vi "Actor Core.vi"(8 "error in":errorcluster, 11 "Main Window in":refnum<class "Main Window.lvclass">) -> (0 "error out":errorcluster, 3 "Actor out":refnum<class "Actor.lvclass">)   [LabVIEW 2023, in "Main Window.lvlib" / "Main Window.lvclass"]
doc: "(<B>Filename</B>: Actor Framework.lvlib:Actor.lvclass:Actor Core.vi)\n\nReceives messages to the actor, reacts to them, and initiates any error handling that may shut the actor down.\n\nDescendant classes may override this VI to append parallel tasks for the actor to complete while it handles messages. Overrides use the Call Parent Method node."
uses:
  Main Window.lvclass
  C:/Program Files/National Instruments/LabVIEW 2023/vi.lib/ActorFramework/Actor/Actor.lvclass
  <vilib>/ActorFramework/Actor/Actor.lvclass
  Resources/Type Defs/Camera Settings.ctl
  Application/Mode.ctl
  Resources/Type Defs/Movie auto-numbering.ctl
  Main Window.lvclass/Main Window.ctl
  <vilib>/ActorFramework/Actor/Actor.lvclass/Actor.ctl
  <vilib>/ActorFramework/Message Enqueuer/Message Enqueuer.lvclass/Message Enqueuer.ctl
  Application Messages/Stop Live Mode Msg/Stop Live Mode Msg.lvclass/Stop Live Mode Msg.ctl
  Application Messages/Set Enabled Cameras Msg/Set Enabled Cameras Msg.lvclass/Set Enabled Cameras Msg.ctl
  Application Messages/Start Live Mode Msg/Start Live Mode Msg.lvclass/Start Live Mode Msg.ctl
  Application Messages/Open Shutter Msg/Open Shutter Msg.lvclass/Open Shutter Msg.ctl
  Hardware/Microscope/ti2lv/ti2_lightPath.ctl
  Application Messages/Set Detection Msg/Set Detection Msg.lvclass/Set Detection Msg.ctl
  Application Messages/Stage Forward Msg/Stage Forward Msg.lvclass/Stage Forward Msg.ctl
  Application Messages/Photobleach Custom Msg/Photobleach Custom Msg.lvclass/Photobleach Custom Msg.ctl
  Application Messages/Set Laser Power Msg/Set Laser Power Msg.lvclass/Set Laser Power Msg.ctl
  Resources/Type Defs/Movie Series.ctl
  Application Messages/Start Recording Msg/Start Recording Msg.lvclass/Start Recording Msg.ctl
  Application Messages/Start Autofocus Msg/Start Autofocus Msg.lvclass/Start Autofocus Msg.ctl
  Application Messages/Stage Enforce Limits Msg/Stage Enforce Limits Msg.lvclass/Stage Enforce Limits Msg.ctl
  <vilib>/ActorFramework/Message Enqueuer/Enqueue.vi
  Application Messages/Shut Down Msg/Shut Down Msg.lvclass
  C:/Program Files/National Instruments/LabVIEW 2023/vi.lib/ActorFramework/Message/Message.lvclass
  Application Messages/Stop Live Mode Msg/Stop Live Mode Msg.lvclass
  Application Messages/Set Enabled Cameras Msg/Set Enabled Cameras Msg.lvclass
  Application Messages/Start Live Mode Msg/Start Live Mode Msg.lvclass
  Application Messages/Close Shutter Msg/Close Shutter Msg.lvclass
  Application Messages/Open Shutter Msg/Open Shutter Msg.lvclass
  Application Messages/Set Detection Msg/Set Detection Msg.lvclass
  Application Messages/Stage Forward Msg/Stage Forward Msg.lvclass
  Application Messages/Stage Back Msg/Stage Back Msg.lvclass
  Application Messages/Stage Next Lane Msg/Stage Next Lane Msg.lvclass
  Application Messages/Stage Previous Lane Msg/Stage Previous Lane Msg.lvclass
  Application Messages/Photobleach Custom Msg/Photobleach Custom Msg.lvclass
  Application Messages/Stage Move Home Msg/Stage Move Home Msg.lvclass
  Application Messages/Stage Set Home Msg/Stage Set Home Msg.lvclass
  Application Messages/Stage Abort Motion Msg/Stage Abort Motion Msg.lvclass
  Application Messages/Set Laser Power Msg/Set Laser Power Msg.lvclass
  Application Messages/Start Recording Msg/Start Recording Msg.lvclass
  Application Messages/Record Button Off Msg/Cancel Operation Msg.lvclass
  Application Messages/Start Autofocus Msg/Start Autofocus Msg.lvclass
  Application Messages/Stage Enforce Limits Msg/Stage Enforce Limits Msg.lvclass
  Application Messages/Calibrate Polarizer Msg/Calibrate Polarizer Msg.lvclass
  Resources/GLOBAL/GLOBAL Time-critical.vi
  <vilib>/ActorFramework/Message Priority Queue/Priority Enqueue.vi
  Resources/GLOBAL/GLOBAL Debug.vi
  <vilib>/Platform/browser.llb/Open URL in Default Browser (string).vi
  UI Window/UI Window.lvclass
  Hardware/Microscope/ti2lv/ti2lv.lvlib
  C:/FlashGordon/Development/User Interface/UI Window/UI Window.lvclass
  C:/FlashGordon/Development/User Interface/Main Window/Main Window.lvclass
  Application/Application.lvlib
panel:
  in  "Auto-Advance":bool
  out "LaserEnabled":bool[](array[boolean])
  out "current settings":T1={"Exposure Time (ms)"=100.0, "Binning"=enum."2x2", "Scan Mode"=-1, "Frames to Acquire"=1000.0, "Pixel Correction"=FALSE, "Frames to Skip"=1, "File Path"=path "", "Duty cycle"=1.0, "ALEX"=FALSE, "Shutter Enable"=[FALSE, TRUE, FALSE, FALSE], "fluidics trigger frame"=0, "Bit Depth"=15, "Image Width (px)"=0, "Image Height (px)"=0, "Horizontal Offset (px)"=0, "Vertical Offset (px)"=0} {"fluidics trigger frame" max=60000 step=1; "Exposure Time (ms)" min=1.0 max=10000.0 step=1.0}
  out "Saving movie":u8(slide) scale=0.0..100.0
  in  "Stop Button":bool
  in  "Tab Control":enum32{"Imaging", "Advanced"}(tab)
  in  "Stage Position":enum32{"Page 1"}(tab)
  out "Stage Map":picture
  in  "Stop Stage":bool
  in  "Set Home":bool
  in  "Go Home":bool
  in  "Move Forward Button":bool
  in  "Move Back Button":bool
  in  "Next Lane Button":bool
  in  "Previous Lane Button":bool
  in  "Photobleach Button":bool
  in  "Camera Settings":enum32{"Page 1"}(tab)
  in  "frame interval unit":u32(ring)=1 items=["ms"=1, "s"=1000, "min"=60000]
  in  "Use Live Exposure":bool
  in  "Live Exposure Time":dbl=200.0 min=1.0 max=1000.0 step=1.0
  in  "Acquisition Period":dbl=10.0 min=0.1 max=10000.0
  in  "Exposure (ms)":dbl=10.0 min=0.1 max=1000.0 step=1.0
  in  "Illumination:":T2(ring)
  in  "Stream Acquisition":enum32{"Page 1"}(tab)
  in  "Lanes:":i32=1 min=1 max=100 step=1
  in  "Fields:":i32=1 min=1 max=100 step=1
  in  "Frames:":dbl=1000.0 min=10.0
  in  "File Path:":path=path "E:/"
  in  "File Name:":string="Stack"
  in  "Acquisition type":T3=enum."Movie series"
  in  "Injection Countdown":bool
  in  "Auto-Focus":bool
  in  "Microscope Settings":enum32{"Page 1"}(tab)
  out "Measured Power:":string
  in  "Detection":u16(ring)=1 items=["Disabled"]
  in  "Active Shutter Button":bool
  in  "Excitation":T4(array[cluster])=[{"Enable"=FALSE, "Name"="Cy2 (473 nm)", "Power"=0.0}, {"Enable"=TRUE, "Name"="Cy3 (532 nm)", "Power"=0.0}, {"Enable"=FALSE, "Name"="Cy5 (640 nm)", "Power"=0.0}, {"Enable"=FALSE, "Name"="Cy7 (721 nm)", "Power"=0.0}]
  in  "Live Viewer Start":bool
  in  "Cancel Movie Button":bool
  in  "Record Movie Button":bool
  in  "Fluidics Settings":enum32{"Page 1"}(tab)
  in  "Trigger on frame number\n(set to zero to disable)":u16
  in  "Advanced Stage Settings":enum32{"Page 1"}(tab)
  in  "Lane separation (mm)":dbl min=0.0 step=0.001
  in  "Forward step (mm)":dbl min=0.0 step=0.001
  in  "Auto-focus":bool
  in  "Enforce software stage limits":bool=TRUE
  in  "Advanced Illumination Settings":enum32{"Page 2"}(tab)
  out "Duty Cycle:":dbl=0.5 min=0.0 max=1.0 step=0.01 format="%#.3g"
  in  "Calibrate Polarizer":bool
  out "Max shutter rate (Hz)":dbl
  in  "Advanced Camera Settings":enum32{"Page 1"}(tab) caption="Tab Control 2"
  in  "Readout Mode":i32(ring)=-1 items=["Auto"=-1]
  in  "Binning":enum16{"1x1", "2x2", "4x4"}(ring)=enum."2x2"
  in  "Discard First Frames":u32=1
  in  "Pixel Correction":enum16{"Live Only", "On", "Off"}(ring)
  in  "Active Cameras":cluster{"Enable":bool, "Name":string}[](array[cluster])
  out "Current Application Mode":T5
  # "Power (mW)"
  # "(Default = 1)"
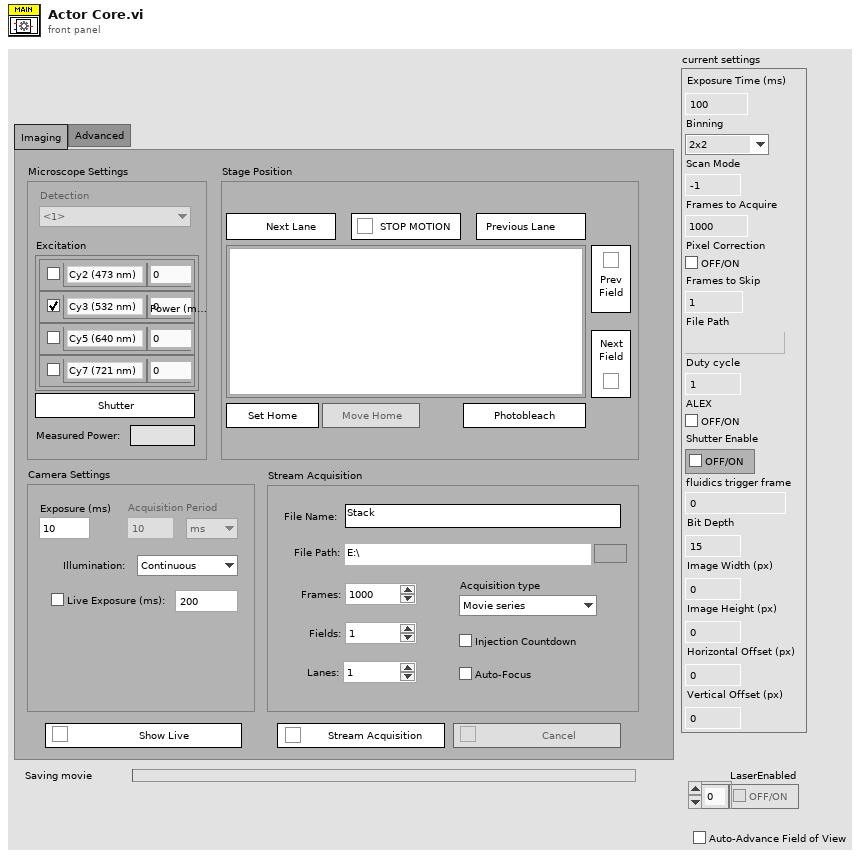
[diagram p1: front panel]
types:
  T1 = typedef "Camera Settings.ctl" = cluster{"Exposure Time (ms)":dbl, "Binning":enum16{"1x1", "2x2", "4x4"}, "Scan Mode":i32, "Frames to Acquire":dbl, "Pixel Correction":bool, "Frames to Skip":u32, "File Path":path, "Duty cycle":dbl, "ALEX":bool, "Shutter Enable":bool[], "fluidics trigger frame":u16, "Bit Depth":u16, "Image Width (px)":u16, "Image Height (px)":u16, "Horizontal Offset (px)":u16, "Vertical Offset (px)":u16}
  T2 = enum16{"Continuous", "Stroboscopic", "Alternating"}
  T3 = typedef "Movie auto-numbering.ctl" = enum16{"Single movie", "Movie series", "Multi-lane series"}
  T4 = cluster{"Enable":bool, "Name":string, "Power":dbl}[]
  T5 = typedef "Application.lvlib/Mode.ctl" = enum16{"Idle", "Cancel", "Live", "Stream", "Autofocus", "Z-Stack"}
  T6 = enum8{"Enabled", "Disabled", "Disabled and Grayed Out"}
  T7 = enum16{"Disable", "Laser Quantum", "Coherent OBIS", "PRM1-Z8", "Coherent HOPS"}
  T8 = typedef "Sync Device Type.ctl" = enum16{"Disabled", "NI DAQ", "Arduino DAQ"}
  T9 = typedef "Physical Camera Assignment.ctl" = cluster{"Channel Name":string, "Serial Number":string, "Flip Vertically":bool, "Flip Horizontally":bool, "wavelength":i16, "photonsPerCount":dbl[]}
  T10 = typedef "Shutter Configuration.ctl" = cluster{"IO Line":tag, "Name":string, "Wavelength":u16, "Max rate (Hz)":dbl}
  T11 = cluster{"Name":string, "Filter Position":u16, "Optical Path":u16}[]
  T12 = typedef "Microscope Type.ctl" = enum16{"Disable", "TE2000", "Eclipse Ti", "Ti2"}
  T13 = enum16{"Disabled", "ESP301", "Ti2", "Ludl", "ASI"}
  T14 = typedef "Laser Configuration.ctl" = cluster{"Serial Port":refnum<visa-resource-name>, "Laser Type":enum16{"Disable", "Laser Quantum", "Coherent OBIS", "PRM1-Z8", "Coherent HOPS", "Cobolt"}, "Polarizer Amplitude":dbl, "Polarizer Theta Zero":dbl, "Wavelength":u16}
  T15 = enum16{"Disable", "Laser Quantum", "Coherent OBIS", "PRM1-Z8", "Coherent HOPS", "Cobolt"}
  T16 = cluster{"Enable":bool, "Name":string, "Power":dbl}
  T17 = typedef "Movie Series.ctl" = cluster{"Camera Settings":T1, "Auto-Advance":bool, "Auto Focus":bool, "Injection Countdown":bool, "Fields":i32, "Lanes":i32, "Acquisition type":T3}
  T18 = typedef "ti2lv.lvlib/ti2_lightPath.ctl" = i32
  T19 = cluster{"Name":string, "Filter Position":u16, "Optical Path":u16}
  T20 = enum16{"Left Button", "Center Button", "Right Button", "Window Close"}
  T21 = cluster{"Enable":bool, "Name":bool, "Power":bool}[]
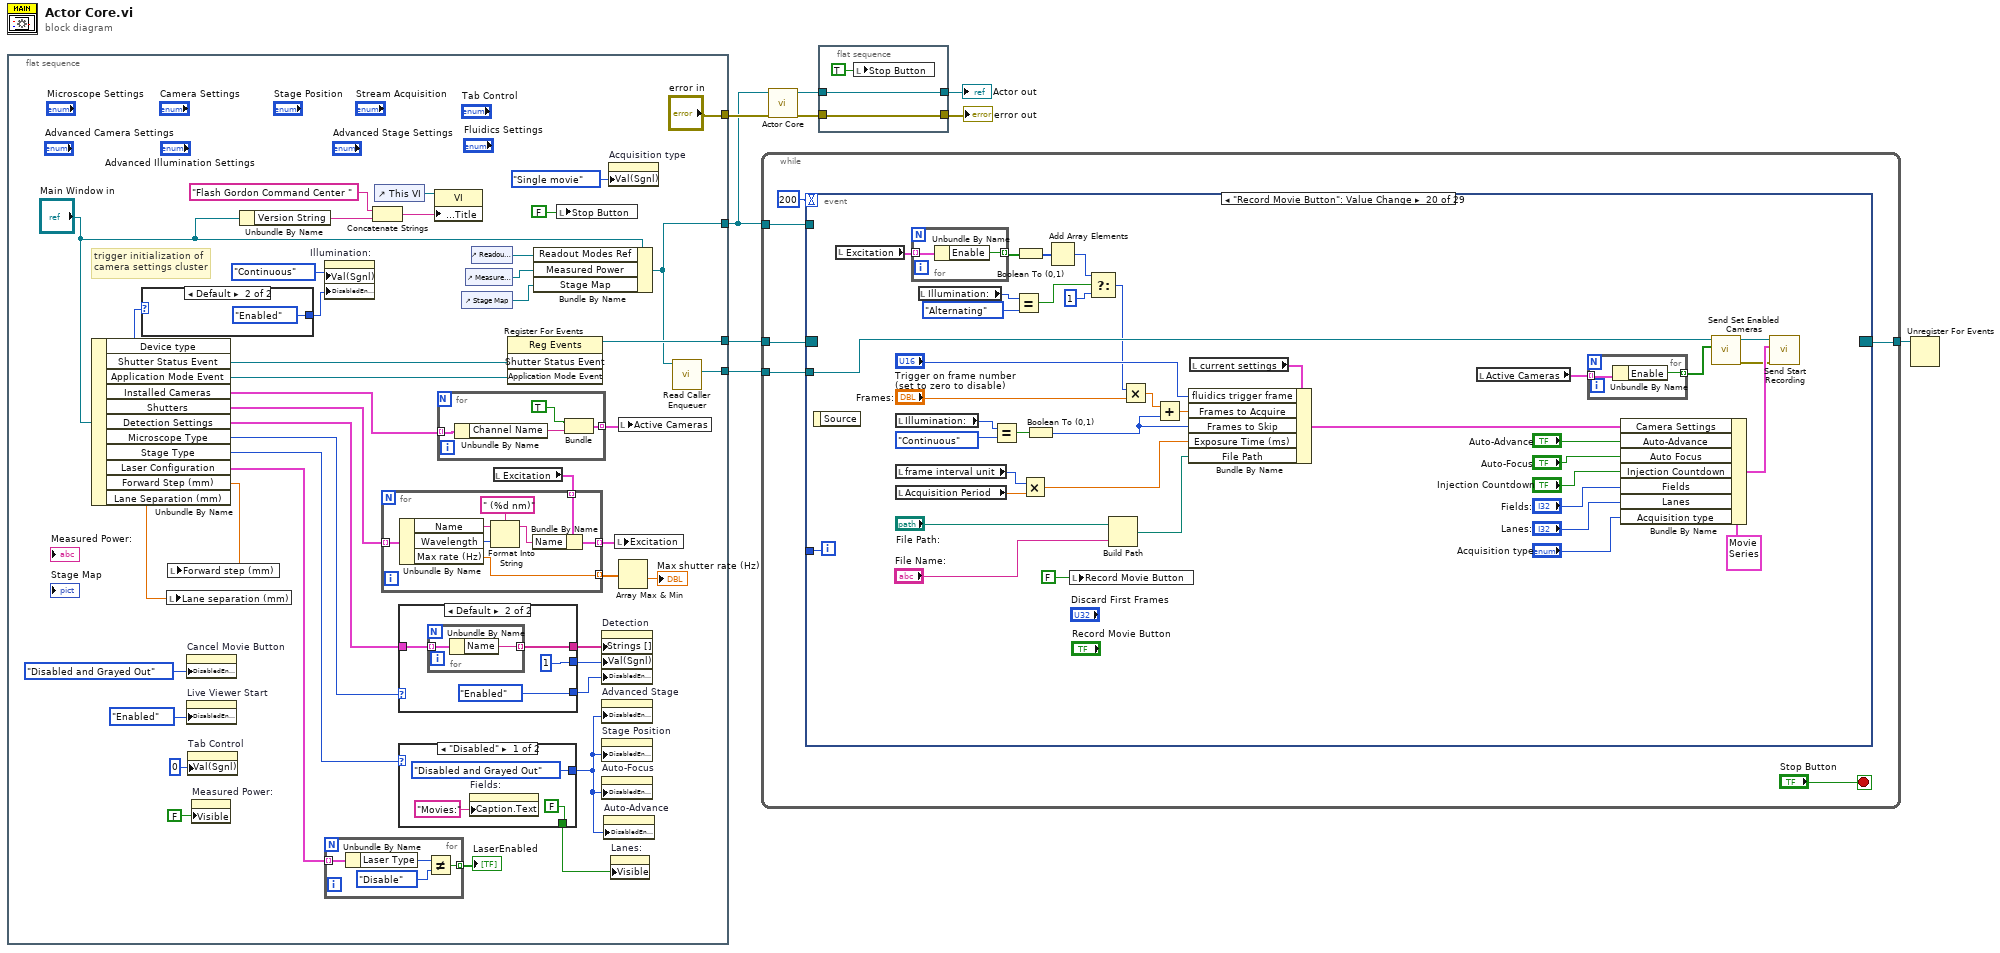
[diagram p0: block diagram]
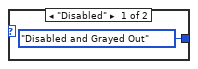
[diagram p2: hidden frame]
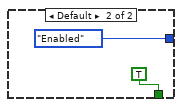
[diagram p3: hidden frame]
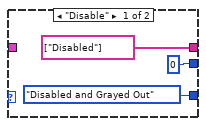
[diagram p4: hidden frame]
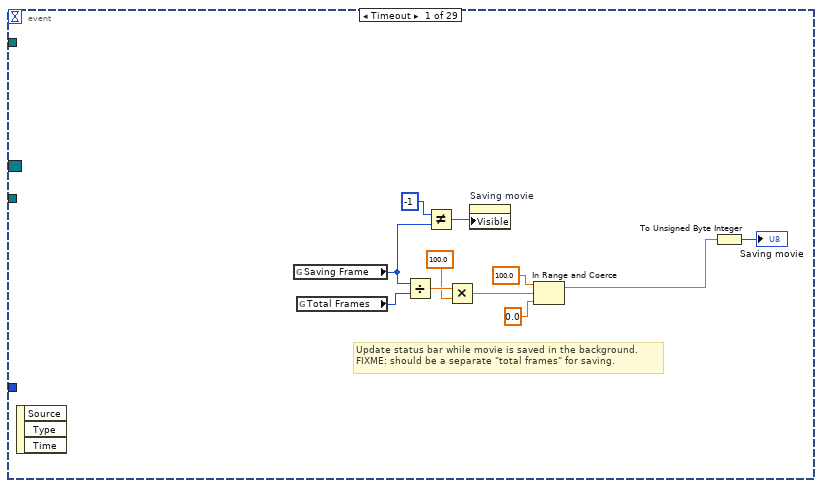
[diagram p5: hidden frame]
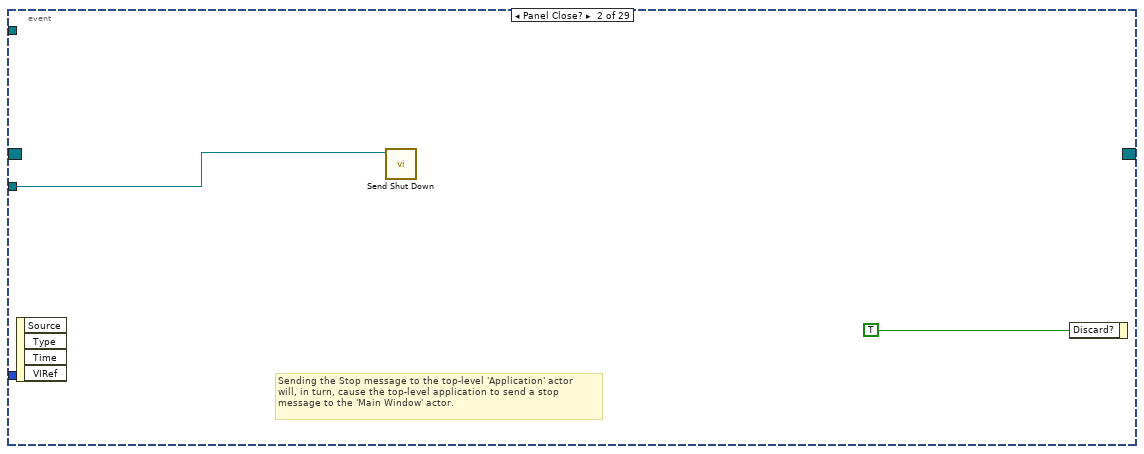
[diagram p6: hidden frame]
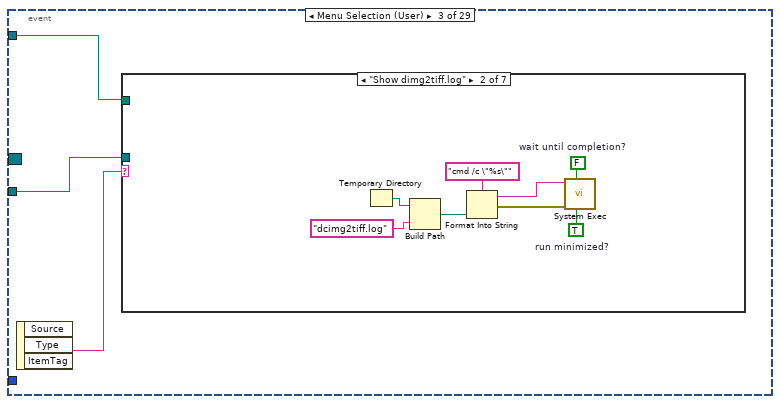
[diagram p7: hidden frame]
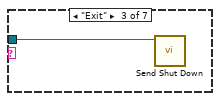
[diagram p9: hidden frame]
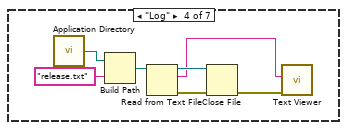
[diagram p10: hidden frame]
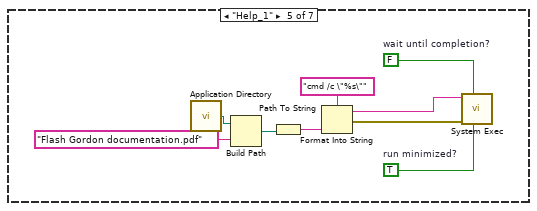
[diagram p11: hidden frame]
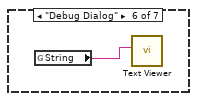
[diagram p12: hidden frame]
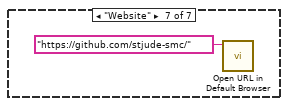
[diagram p13: hidden frame]
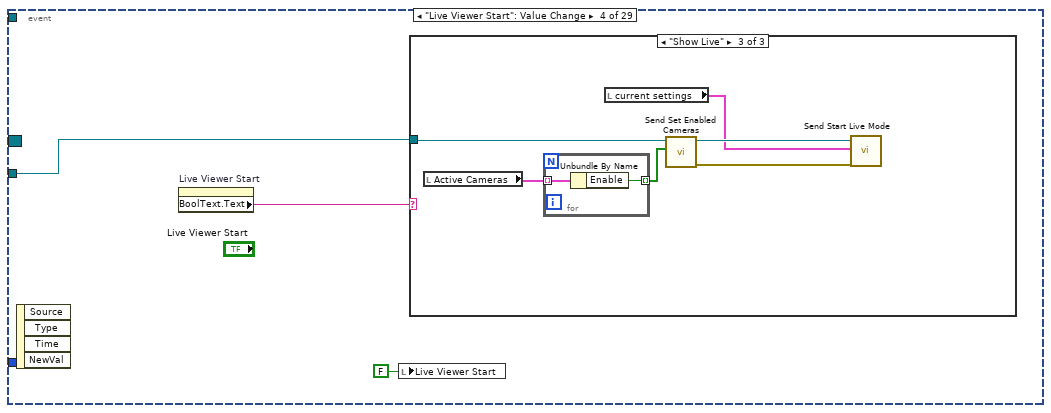
[diagram p14: hidden frame]
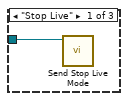
[diagram p15: hidden frame]
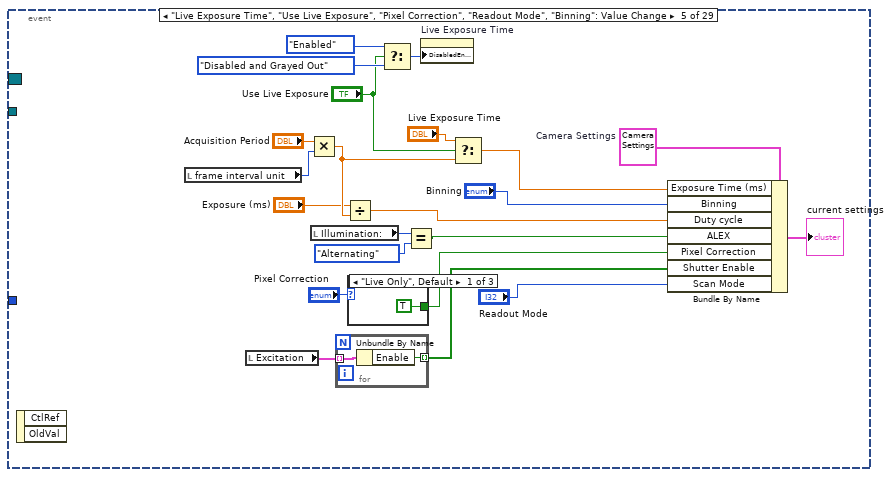
[diagram p17: hidden frame]
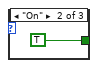
[diagram p18: hidden frame]
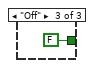
[diagram p19: hidden frame]
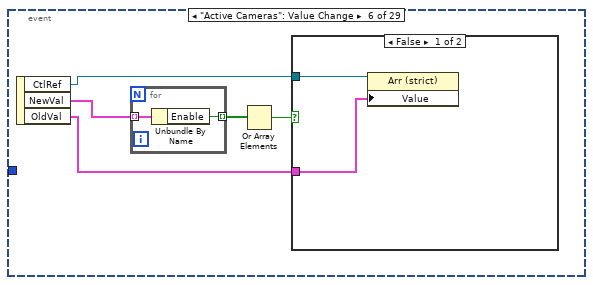
[diagram p20: hidden frame]
diagram:
  n1 = flat-sequence {
    tunnel: [w28] -> w7
    tunnel: ["error in"] -> w8
    tunnel: [w42] -> w6
    tunnel: [w41] -> w5
    frame #0 {
      # "trigger initialization of\ncamera settings cluster"
      n2 = Unbundle By Name("Main Window in") -> ("Device type"=w16:T8, "Shutter Status Event"=w32:refnum<user-event>, "Application Mode Event"=w35:refnum<user-event>, "Installed Cameras"=w23:T9[], "Shutters"=w24:T10[], "Detection Settings"=w37:T11, "Microscope Type"=w40:T12, "Stage Type"=w25:T13, "Laser Configuration"=w20:T14[], "Forward Step (mm)"=w14:dbl, "Lane Separation (mm)"=w13:dbl)
      n3 = case shown="Default" w16 {
        tunnel: [T6."Disabled and Grayed Out" ("Disabled") T6."Enabled" ("Disabled")] -> w15
        frame "Disabled" {
        }
        frame Default {
        }
      }
      n4 = local write "Lane separation (mm)"(w13) -> ()
      n5 = local write "Forward step (mm)"(w14) -> ()
      n6 = property on="Cancel Movie Button" class="Bool (strict)"("DisabledEnum"=T6."Disabled and Grayed Out" ("Disabled")) -> ()  [unwired: 2 in, 2 out]
      n7 = property on="Live Viewer Start" class="Bool (strict)"("DisabledEnum"=T6."Enabled" ("Disabled")) -> ()  [unwired: 2 in, 2 out]
      n8 = property on="Tab Control" class="TabCtl (strict)"("Val(Sgnl)"=0) -> ()  [unwired: 2 in, 2 out]
      n9 = property on="Measured Power:" class="Str"("Visible"=FALSE) -> ()  [unwired: 2 in, 2 out]
      n10 = Unbundle By Name("Main Window in") -> ("Version String"=w47:string)
      n11 = property on="Illumination:" class="Enum (strict)"("Val(Sgnl)"=T2."Continuous" ("Value (Signaling)"), "DisabledEnum"=w15) -> ()  [unwired: 2 in, 2 out]
      n12 = for {
        tunnel: w20 -> [w57] mode=indexing
        tunnel: [w55] -> w19 mode=indexing
        n13 = Unbundle By Name(w57) -> ("Laser Type"=w56:T15)
        n14 = Not Equal?(x=w56, y=T7."Disable") -> (x != y?=w55:bool)
      }
      "LaserEnabled" <- w19
      n15 = Concatenate Strings("Flash Gordon Command Center " ("Front Panel Window:Title"), w47) -> (w48:string)
      n16 = control-ref of="This VI"() -> (w49:refnum<vi>)
      n17 = case shown="Default" w40 {
        tunnel: [T6."Disabled and Grayed Out" ("Disabled") T6."Enabled" ("Disabled")] -> w39
        tunnel: [string[] ["Disabled"] w68] -> w38
        tunnel: w37 -> [_ w67]
        tunnel: [u16 0 u16 1] -> w36
        frame "Disable" {
        }
        frame Default {
          n18 = for {
            tunnel: w67 -> [w71] mode=indexing
            tunnel: [w70] -> w68 mode=indexing
            n19 = Unbundle By Name(w71) -> ("Name"=w70:string)
          }
        }
      }
      n20 = case shown="\"Disabled\"" w25 {
        tunnel: [T6."Disabled and Grayed Out" ("Disabled") T6."Enabled" ("Disabled")] -> w12
        tunnel: [FALSE TRUE] -> w11
        frame "Disabled" {
          n21 = property on="Fields:" class="DigNum (strict)"("Caption.Text"="Movies:") -> ()  [unwired: 2 in, 2 out]
        }
        frame Default {
        }
      }
      n22 = property class="VI"(reference=w49, "Front Panel.Title"=w48) -> ()  [unwired: 1 in, 2 out]
      n23 = for {
        tunnel: w23 -> [w83] mode=indexing
        tunnel: [w81] -> w30 mode=indexing
        n24 = Unbundle By Name(w83) -> ("Channel Name"=w82:string)
        n25 = Bundle(TRUE, "Channel Name"=w82) -> (w81:cluster{bool, "Channel Name":string})  [unwired: 1 in]
      }
      n26 = control-ref of="Stage Map"() -> (w17:refnum<vi>)
      n27 = control-ref of="Measured Power:"() -> (w18:refnum<vi>)
      n28 = control-ref of="Readout Mode"() -> (w26:refnum<vi>)
      n29 = local read "Excitation"() -> (w33:T4)
      n30 = for {
        tunnel: w24 -> [w79] mode=indexing
        tunnel: w33 -> [w75] mode=indexing
        tunnel: [w73] -> w43 mode=indexing
        tunnel: [w72] -> w22 mode=indexing
        n31 = Unbundle By Name(w79) -> ("Name"=w78:string, "Wavelength"=w77:u16, "Max rate (Hz)"=w72:dbl)
        n32 = Format Into String(format string=" (%d nm)", initial string=w78, w77) -> (resulting string=w74:string)  [unwired: 1 in, 1 out]
        n33 = Bundle By Name(cluster=w75, "Name"=w74) -> (w73:T16)
      }
      n34 = register-events(w32, w35) -> (reference out=w42:refnum<event-registration>)  [unwired: 2 in, 1 out]
      n35 = Bundle By Name(cluster="Main Window in", "Readout Modes Ref"=w26, "Measured Power"=w18, "Stage Map"=w17) -> (w28:refnum<class "Main Window.lvclass">)
      n36 = local write "Stop Button"(FALSE ("Stop Button")) -> ()
      n37 = property on="Detection" class="Ring (strict)"("Strings []"=w38, "Val(Sgnl)"=w36, "DisabledEnum"=w39) -> ()  [unwired: 2 in, 2 out]
      n38 = property on="Advanced Stage" class="TabCtl (strict)"("DisabledEnum"=w12) -> ()  [unwired: 2 in, 2 out]
      n39 = property on="Stage Position" class="TabCtl (strict)"("DisabledEnum"=w12) -> ()  [unwired: 2 in, 2 out]
      n40 = property on="Auto-Focus" class="Bool (strict)"("DisabledEnum"=w12) -> ()  [unwired: 2 in, 2 out]
      n41 = property on="Auto-Advance" class="Bool (strict)"("DisabledEnum"=w12) -> ()  [unwired: 2 in, 2 out]
      n42 = property on="Acquisition type" class="Enum (strict)"("Val(Sgnl)"=Movie_auto-numbering."Single movie" ("Value (Signaling)")) -> ()  [unwired: 2 in, 2 out]
      n43 = property on="Lanes:" class="DigNum (strict)"("Visible"=w11) -> ()  [unwired: 2 in, 2 out]
      n44 = local write "Excitation"(w43) -> ()
      n45 = local write "Active Cameras"(w30) -> ()
      n46 = Array Max & Min(array=w22) -> (min value=→"Max shutter rate (Hz)":dbl)  [unwired: 3 out]
      n47 = call <vilib>:"Read Caller Enqueuer.vi"("Actor"=w28) -> ("Caller Enqueuer"=w41:refnum<class "Message Enqueuer.lvclass">)  [unwired: 10 in]
    }
  }
  n48 = while {
    tunnel: w5 -> [w90]
    tunnel: w6 -> [w89]
    tunnel: [w87] -> w9
    tunnel: w7 -> [w86]
    i -> [w88]
    stop <- "Stop Button" stop-if-true
    n49 = event shown="[19] \"Record Movie Button\": Value Change" {
      selector: w89 -> [_ _ _ _ _ _ _ _ _ _ _ _ _ _ _ _ _ _ _ _ _ _ _ _ _ _ _ _ _]
      dyn-events: [_ _ _ _ _ _ _ _ _ _ _ _ _ _ _ _ _ _ _ _ _ _ _ _ _ _ _ _ _] -> w87
      timeout: 200 -> [_ _ _ _ _ _ _ _ _ _ _ _ _ _ _ _ _ _ _ _ _ _ _ _ _ _ _ _ _]
      tunnel: w90 -> [_ w103 w105 w136 _ _ _ w192 w213 w224 w226 w228 w229 w237 _ w251 w255 w259 w278 w355 _ _ w381 _ _ _ w433 w441 w442]
      tunnel: w88 -> [_ _ _ _ _ _ _ _ _ _ _ _ _ _ _ _ _ _ _ _ _ _ _ _ _ _ _ _ _]
      tunnel: w86 -> [_ _ w104 _ _ _ _ _ w212 _ _ _ _ _ _ _ _ _ w271 _ _ _ _ _ _ _ _ _ _]
      event Timeout {
        # "Update status bar while movie is saved in the background.\nFIXME: should be a separate \"total frames\" for saving."
        n50 = event-data() -> ()  [unwired: 1 in, 3 out]
        n51 = global read "GLOBAL Time-critical.vi" "Saving Frame"() -> (w92:i32)
        n52 = global read "GLOBAL Time-critical.vi" "Total Frames"() -> (w94:i32)
        n53 = Divide(x=w92, y=w94) -> (x/y=w98:dbl)
        n54 = Not Equal?(x=-1, y=w92) -> (x != y?=w93:bool)
        n55 = Multiply(x=w98, y=100.0) -> (x*y=w100:dbl)
        n56 = property on="Saving movie" class="Slide (strict)"("Visible"=w93) -> ()  [unwired: 2 in, 2 out]
        n57 = In Range and Coerce(upper limit=100.0, x=w100, lower limit=0.0) -> (coerced(x)=w101:dbl)  [unwired: 1 out]
        n58 = To Unsigned Byte Integer(number=w101) -> (unsigned 8bit integer=→"Saving movie":u8)
      }
      event Panel Close? {
        # "Sending the Stop message to the top-level 'Application' actor\nwill, in turn, cause the top-level application to send a stop \nmessage to the 'Main Window' actor."
        n59 = event-data() -> ()  [unwired: 1 in, 4 out]
        n60 = call "Send Shut Down.vi"("Message Enqueuer"=w103) -> ()  [unwired: 9 in, 2 out]
        n61 = event-data("Discard?"=TRUE) -> ()  [unwired: 1 in, 1 out]
      }
      event Menu Selection (User) {
        n62 = event-data() -> ("ItemTag"=w106:string)  [unwired: 1 in, 2 out]
        n63 = case shown="\"Show dimg2tiff.log\"" w106 {
          tunnel: w105 -> [_ _ w115 _ _ _ _]
          tunnel: w104 -> [_ _ _ _ _ _ _]
          frame Default {
          }
          frame "Show dimg2tiff.log" {
            w112 = TRUE  # run minimized?
            w111 = FALSE  # wait until completion?
            n64 = Temporary Directory() -> (w109:path)
            n65 = Build Path(base path=w109, name or relative path="dcimg2tiff.log") -> (appended path=w107:path)
            n66 = Format Into String(format string="cmd /c \"%s\"", w107) -> (resulting string=w110:string, error out=w114:errorcluster)  [unwired: 2 in]
            n67 = call <vilib>:"System Exec.vi"("run minimized? (F)"=w112, "wait until completion? (T)"=w111, "error in (no error)"=w114, "command line"=w110) -> ()  [unwired: 4 in, 4 out]
          }
          frame "Exit" {
            n68 = call "Send Shut Down.vi"("Message Enqueuer"=w115) -> ()  [unwired: 9 in, 2 out]
          }
          frame "Log" {
            n69 = call <vilib>:"Application Directory.vi"() -> ("Application Directory"=w118:path)
            n70 = Build Path(base path=w118, name or relative path="release.txt") -> (appended path=w121:path)
            n71 = Read from Text File(file (use dialog)=w121) -> (refnum out=w122:refnum<file>, text=w117:string, error out=w119:errorcluster)  [unwired: 3 in, 1 out]
            n72 = Close File(refnum=w122, error in=w119) -> (error out=w116:errorcluster)  [unwired: 1 out]
            n73 = call "Text Viewer.vi"("error in"=w116, "Change Log Display"=w117) -> ()  [unwired: 9 in, 1 out]
          }
          frame "Help_1" {
            w125 = TRUE  # run minimized?
            w124 = FALSE  # wait until completion?
            n74 = call <vilib>:"Application Directory.vi"() -> ("Application Directory"=w129:path)
            n75 = Build Path(base path=w129, name or relative path="Flash Gordon documentation.pdf") -> (appended path=w130:path)
            n76 = Path To String(path=w130) -> (string=w131:string)
            n77 = Format Into String(format string="cmd /c \"%s\"", w131) -> (resulting string=w123:string, error out=w128:errorcluster)  [unwired: 2 in]
            n78 = call <vilib>:"System Exec.vi"("run minimized? (F)"=w125, "wait until completion? (T)"=w124, "error in (no error)"=w128, "command line"=w123) -> ()  [unwired: 4 in, 4 out]
          }
          frame "Debug Dialog" {
            n79 = global read "GLOBAL Debug.vi" "String"() -> (w132:string)
            n80 = call "Text Viewer.vi"("Change Log Display"=w132) -> ()  [unwired: 10 in, 1 out]
          }
          frame "Website" {
            n81 = call-poly <vilib>:"Open URL in Default Browser.vi"("URL"="https://github.com/stjude-smc/") -> ()  [unwired: 5 in, 2 out]
          }
        }
      }
      event "Live Viewer Start": Value Change {
        n82 = event-data() -> ()  [unwired: 1 in, 4 out]
        n83 = property on="Live Viewer Start" class="Bool (strict)"() -> ("BoolText.Text"=w135:string)  [unwired: 2 in, 2 out]
        n84 = local write "Live Viewer Start"(FALSE ("Live Viewer Start")) -> ()
        n85 = case shown="\"Show Live\"" w135 {
          tunnel: w136 -> [w137 _ w141]
          frame "Stop Live" {
            n86 = call "Send Stop Live Mode.vi"("Message Enqueuer"=w137) -> ()  [unwired: 9 in, 2 out]
          }
          frame Default {
          }
          frame "Show Live" {
            n87 = local read "Active Cameras"() -> (w143:cluster{"Enable":bool, "Name":string}[])
            n88 = for {
              tunnel: w143 -> [w145] mode=indexing
              tunnel: [w144] -> w142 mode=indexing
              n89 = Unbundle By Name(w145) -> ("Enable"=w144:bool)
            }
            n90 = local read "current settings"() -> (w138:T1)
            n91 = call "Send Set Enabled Cameras.vi"("Cameras Enabled"=w142, "Message Enqueuer"=w141) -> ("error out"=w139:errorcluster, "Message Enqueuer out"=w140:refnum<class "Message Enqueuer.lvclass">)  [unwired: 8 in]
            n92 = call "Send Start Live Mode.vi"("error in (no error)"=w139, "Camera Settings"=w138, "Message Enqueuer"=w140) -> ()  [unwired: 7 in, 2 out]
          }
        }
      }
      event "Live Exposure Time", "Use Live Exposure", "Pixel Correction", "Readout Mode", "Binning": Value Change {
        w158 = T1 {"Exposure Time (ms)"=100.0, "Binning"=enum."2x2", "Scan Mode"=0, "Frames to Acquire"=1000.0, "Pixel Correction"=FALSE, "Frames to Skip"=0, "File Path"=path "", "Duty cycle"=0.0, "ALEX"=FALSE, "Shutter Enable"=[], "fluidics trigger frame"=0, "Bit Depth"=0, "Image Width (px)"=0, "Image Height (px)"=0, "Horizontal Offset (px)"=0, "Vertical Offset (px)"=0}  # Camera Settings
        n93 = event-data() -> ()  [unwired: 1 in, 2 out]
        n94 = local read "frame interval unit"() -> (w164:u32)
        n95 = local read "Excitation"() -> (w156:T4)
        n96 = Multiply(x="Acquisition Period", y=w164) -> (x*y=w162:dbl)
        n97 = local read "Illumination:"() -> (w150:T2)
        n98 = for {
          tunnel: w156 -> [w169] mode=indexing
          tunnel: [w168] -> w155 mode=indexing
          n99 = Unbundle By Name(w169) -> ("Enable"=w168:bool)
        }
        n100 = Divide(x="Exposure (ms)", y=w162) -> (x/y=w163:dbl)
        n101 = case shown="\"Live Only\", Default" "Pixel Correction" {
          tunnel: [TRUE ("Pixel Correction (Flash)") TRUE ("Pixel Correction (Flash)") FALSE ("Pixel Correction (Flash)")] -> w148
          frame "Live Only", Default {
          }
          frame "On" {
          }
          frame "Off" {
          }
        }
        n102 = Select(t=T6."Enabled" ("Disabled"), s="Use Live Exposure", f=T6."Disabled and Grayed Out" ("Disabled")) -> (s? t:f=w165:T6)
        n103 = Equal?(x=w150, y=T2."Alternating") -> (x = y?=w147:bool)
        n104 = property on="Live Exposure Time" class="DigNum (strict)"("DisabledEnum"=w165) -> ()  [unwired: 2 in, 2 out]
        n105 = Select(t="Live Exposure Time", s="Use Live Exposure", f=w162) -> (s? t:f=w157:dbl)
        n106 = Bundle By Name(cluster=w158, "Exposure Time (ms)"=w157, "Binning"="Binning", "Duty cycle"=w163, "ALEX"=w147, "Pixel Correction"=w148, "Shutter Enable"=w155, "Scan Mode"="Readout Mode") -> (→"current settings":T1)
      }
      event "Active Cameras": Value Change {
        n107 = event-data() -> ("CtlRef"=w174:refnum<vi>, "NewVal"=w177:cluster{"Enable":bool, "Name":string}[], "OldVal"=w173:cluster{"Enable":bool, "Name":string}[])  [unwired: 1 in]
        n108 = for {
          tunnel: w177 -> [w181] mode=indexing
          tunnel: [w180] -> w176 mode=indexing
          n109 = Unbundle By Name(w181) -> ("Enable"=w180:bool)
        }
        n110 = Or Array Elements(Boolean array=w176) -> (logical OR=w175:bool)
        n111 = case shown="False" w175 {
          tunnel: w174 -> [w179 _]
          tunnel: w173 -> [w178 _]
          frame False {
            n112 = property class="Arr (strict)"(reference=w179, "Value"=w178) -> ()  [unwired: 1 in, 2 out]
          }
          frame True {
          }
        }
      }
      event "frame interval unit": Value Change {
        n113 = event-data() -> ("OldVal"=w183:u32, "NewVal"=w182:u32)  [unwired: 1 in, 4 out]
        n114 = local read "Acquisition Period"() -> (w185:dbl)
        n115 = Multiply(x=w185, y=w183) -> (x*y=w184:dbl)
        n116 = Divide(x=w184, y=w182) -> (x/y=w186:dbl)
        n117 = local write "Acquisition Period"(w186) -> ()
      }
      event "Active Shutter Button": Value Change {
        n118 = event-data() -> ()  [unwired: 1 in, 6 out]
        n119 = local read "Excitation"() -> (w191:T4)
        n120 = local read "Illumination:"() -> (w189:T2)
        n121 = for {
          tunnel: w191 -> [w195] mode=indexing
          tunnel: [w194] -> w190 mode=indexing
          n122 = Unbundle By Name(w195) -> ("Enable"=w194:bool)
        }
        n123 = Equal?(x=w189, y=T2."Alternating") -> (x = y?=w187:bool)
        n124 = case shown="True" "Active Shutter Button" {
          tunnel: w192 -> [w196 w199]
          tunnel: w190 -> [_ w198]
          tunnel: w187 -> [_ w197]
          frame False {
            n125 = call "Send Close Shutter.vi"("Message Enqueuer"=w196) -> ()  [unwired: 9 in, 2 out]
          }
          frame True {
            n126 = call "Send Open Shutter.vi"("ALEX?"=w197, "Array"=w198, "Message Enqueuer"=w199) -> ()  [unwired: 7 in, 2 out]
          }
        }
      }
      event "Detection": Value Change {
        w204 = T18 1 items=["Eyepieces"=1, "Right"=2, "Bottom"=3, "Left"=4] ("Optical Path")
        n127 = event-data() -> ("OldVal"=w206:u16)  [unwired: 1 in, 5 out]
        n128 = Unbundle By Name(w212) -> ("Detection Settings"=w211:T11)
        n129 = local read "Excitation"() -> (w208:T4)
        n130 = Index Array(array=w211, index="Detection") -> (element=w210:T19)
        n131 = for {
          tunnel: w208 -> [w217] mode=indexing
          tunnel: [w215] -> w207 mode=indexing
          n132 = Unbundle By Name(w217) -> ("Power"=w216:dbl)
          n133 = Greater?(x=w216, y=20.0) -> (0:w215:bool)
        }
        n134 = Unbundle By Name(w210) -> ("Filter Position"=w209:u16, "Optical Path"=w205:u16)
        n135 = Equal?(x=w205, y=w204) -> (x = y?=w202:bool)
        n136 = Or Array Elements(Boolean array=w207) -> (logical OR=w201:bool)
        n137 = And(x=w202, y=w201) -> (x .and. y?=w203:bool)
        n138 = case shown="True" w203 {
          tunnel: w213 -> [w220 _]
          tunnel: w209 -> [w219 _]
          tunnel: w205 -> [w218 _]
          tunnel: w206 -> [_ w221]
          frame False {
            n139 = call "Send Set Detection.vi"("Optical Path"=w218, "Filter Position"=w219, "Message Enqueuer"=w220) -> ()  [unwired: 7 in, 2 out]
          }
          frame True {
            n140 = property on="Detection" class="Ring (strict)"("Value"=w221) -> ()  [unwired: 2 in, 2 out]
            n141 = One Button Dialog(message="Laser power unsafe") -> ()  [unwired: 1 in, 1 out]
          }
        }
      }
      event "Move Forward Button": Value Change {
        n142 = event-data() -> ()  [unwired: 1 in, 6 out]
        n143 = call "Send Stage Forward.vi"("Message Enqueuer"=w224) -> ()  [unwired: 9 in, 2 out]
        n144 = local write "Move Forward Button"(FALSE ("Move Forward Button")) -> ()
      }
      event "Move Back Button": Value Change {
        n145 = event-data() -> ()  [unwired: 1 in, 6 out]
        n146 = call "Send Stage Back.vi"("Message Enqueuer"=w226) -> ()  [unwired: 9 in, 2 out]
        n147 = local write "Move Back Button"(FALSE ("Move Back Button")) -> ()
      }
      event "Next Lane Button": Value Change {
        n148 = event-data() -> ()  [unwired: 1 in, 6 out]
        n149 = call "Send Stage Next Lane.vi"("Message Enqueuer"=w228) -> ()  [unwired: 9 in, 2 out]
        n150 = local write "Next Lane Button"(FALSE ("Next Lane Button")) -> ()
      }
      event "Previous Lane Button": Value Change {
        n151 = event-data() -> ()  [unwired: 1 in, 6 out]
        n152 = call "Send Stage Previous Lane.vi"("Message Enqueuer"=w229) -> ()  [unwired: 9 in, 2 out]
      }
      event "Photobleach Button": Value Change {
        n153 = event-data() -> ()  [unwired: 1 in, 6 out]
        n154 = local read "Excitation"() -> (w231:T4)
        n155 = local write "Photobleach Button"(FALSE ("Photobleach Button")) -> ()
        n156 = for {
          tunnel: w231 -> [w239] mode=indexing
          tunnel: [w238] -> w230 mode=indexing
          n157 = Unbundle By Name(w239) -> ("Enable"=w238:bool)
        }
        n158 = call <vilib>:"Three Button Dialog.vi"("Center Button Text (\"No\")"="Custom Length..." ("Center Button Text (\"No\")"), "Left Button Text (\"Yes\")"="OK" ("Left Button Text (\"Yes\")"), "message"="Please confirm that prism is positioned at the far end of the lane. \nOtherwise microscope WILL BE DAMAGED.") -> ("Which Button?"=w233:T20)  [unwired: 8 in]
        n159 = case shown="\"Center Button\"" w233 {
          tunnel: w237 -> [w241 w244 _]
          tunnel: w230 -> [w240 w243 _]
          frame "Left Button", Default {
            n160 = call "Send Photobleach Custom.vi"("Shutter Enable"=w240, "Length (mm)"=0.0, "Message Enqueuer"=w241) -> ()  [unwired: 7 in, 2 out]
          }
          frame "Center Button" {
            n161 = call "Custom Photobleach Length.vi"() -> ("Canceled"=w245:bool, "Length (mm)"=w246:dbl)  [unwired: 10 in]
            n162 = case shown="False" w245 {
              tunnel: w246 -> [w249 _]
              tunnel: w244 -> [w248 _]
              tunnel: w243 -> [w247 _]
              frame False {
                n163 = call "Send Photobleach Custom.vi"("Shutter Enable"=w247, "Length (mm)"=w249, "Message Enqueuer"=w248) -> ()  [unwired: 7 in, 2 out]
              }
              frame True {
              }
            }
          }
          frame "Right Button" {
          }
        }
      }
      event User Event {
        n164 = event-data() -> ("Shutters Active?"=w250:bool)  [unwired: 1 in, 4 out]
        n165 = property on="Active Shutter Button" class="Bool (strict)"("Value"=w250) -> ()  [unwired: 2 in, 2 out]
      }
      event "Go Home": Value Change {
        n166 = event-data() -> ()  [unwired: 1 in, 6 out]
        n167 = local write "Go Home"(FALSE ("Go Home")) -> ()
        n168 = call "Send Stage Move Home.vi"("Message Enqueuer"=w251) -> ()  [unwired: 9 in, 2 out]
      }
      event "Set Home": Value Change {
        n169 = event-data() -> ()  [unwired: 1 in, 6 out]
        n170 = local write "Set Home"(FALSE ("Set Home")) -> ()
        n171 = Two Button Dialog(message="Please confirm that prism is positioned at \nthe far end of the lane before proceeding.") -> (T button?=w253:bool)  [unwired: 2 in]
        n172 = case shown="True" w253 {
          tunnel: w255 -> [_ w258]
          frame False {
          }
          frame True {
            n173 = call "Send Stage Set Home.vi"("Message Enqueuer"=w258) -> ()  [unwired: 9 in, 2 out]
            n174 = property on="Go Home" class="Bool (strict)"("DisabledEnum"=T6."Enabled" ("Disabled")) -> ()  [unwired: 2 in, 2 out]
          }
        }
      }
      event "Stop Stage": Value Change {
        n175 = event-data() -> ()  [unwired: 1 in, 6 out]
        n176 = local write "Stop Stage"(FALSE ("Stop Stage")) -> ()
        n177 = call "Send Stage Abort Motion.vi"("Message Enqueuer"=w259) -> ()  [unwired: 9 in, 2 out]
      }
      event "Excitation": Value Change {
        w269 = T18 1 items=["Eyepieces"=1, "Right"=2, "Bottom"=3, "Left"=4] ("Optical Path")
        n178 = event-data() -> ("OldVal"=w265:T4)  [unwired: 1 in]
        n179 = Unbundle By Name(w271) -> ("Detection Settings"=w274:T11)
        n180 = local read "Detection"() -> (w272:u16)
        n181 = local read "Illumination:"() -> (w264:T2)
        n182 = local read "Active Shutter Button"() -> (w279:bool)
        n183 = for {
          tunnel: "Excitation" -> [w313] mode=indexing
          tunnel: [w312] -> w275 mode=indexing
          n184 = Unbundle By Name(w313) -> ("Enable"=w312:bool)
        }
        n185 = Not Equal?(x=w265, y="Excitation") -> (x != y?=w268:T21)
        n186 = Index Array(array=w274, index=w272) -> (element=w273:T19)
        n187 = Equal?(x=w264, y=T2."Alternating") -> (x = y?=w262:bool)
        n188 = Unbundle By Name(w273) -> ("Optical Path"=w270:u16)
        n189 = local read "current settings"() -> (w277:T1)
        n190 = local read "LaserEnabled"() -> (w261:bool[])
        n191 = case shown="True" w279 {
          tunnel: w275 -> [_ w316]
          tunnel: w278 -> [_ w315]
          tunnel: w262 -> [_ w314]
          frame False {
          }
          frame True {
            n192 = call "Send Open Shutter.vi"("ALEX?"=w314, "Array"=w316, "Message Enqueuer"=w315) -> ()  [unwired: 7 in, 2 out]
          }
        }
        n193 = Bundle By Name(cluster=w277, "Shutter Enable"=w275) -> (w276:T1)
        n194 = Equal?(x=w270, y=w269) -> (x = y?=w266:bool)
        n195 = local write "current settings"(w276) -> ()
        n196 = for {
          tunnel: w278 -> [w292]
          tunnel: w268 -> [w286] mode=indexing
          tunnel: "Excitation" -> [w285] mode=indexing
          tunnel: w266 -> [w283]
          tunnel: w265 -> [w281]
          tunnel: w261 -> [w280] mode=indexing
          i -> [w293]
          n197 = Unbundle By Name(w285) -> ("Power"=w288:dbl)
          n198 = Cluster To Array(cluster=w286) -> (array=w291:bool[])
          n199 = Index Array(array=w291, index=2) -> (element=w287:bool)
          n200 = Greater?(x=w288, y=20.0) -> (0:w284:bool)
          n201 = And(x=w284, y=w283) -> (x .and. y?=w282:bool)
          n202 = case shown="True" w287 {
            tunnel: w293 -> [_ w297]
            tunnel: w288 -> [_ w298]
            tunnel: w292 -> [_ w299]
            tunnel: w282 -> [_ w296]
            tunnel: w281 -> [_ w295]
            tunnel: w280 -> [_ w294]
            frame False {
            }
            frame True {
              # "Laser power changed"
              n203 = case shown="False" w296 {
                tunnel: w299 -> [w304 _]
                tunnel: w298 -> [w303 _]
                tunnel: w297 -> [w302 _]
                tunnel: w295 -> [w300 w310]
                tunnel: w294 -> [w301 _]
                frame False {
                  n204 = case shown="True" w301 {
                    tunnel: w304 -> [_ w309]
                    tunnel: w303 -> [_ w308]
                    tunnel: w302 -> [_ w307]
                    tunnel: w300 -> [w305 _]
                    frame False {
                      n205 = local write "Excitation"(w305) -> ()
                      n206 = One Button Dialog(message="Laser line not configured") -> ()  [unwired: 1 in, 1 out]
                    }
                    frame True {
                      n207 = call "Send Set Laser Power.vi"("Power"=w308, "laser index"=w307, "Message Enqueuer"=w309) -> ()  [unwired: 7 in, 2 out]
                    }
                  }
                }
                frame True {
                  n208 = local write "Excitation"(w310) -> ()
                  n209 = One Button Dialog(message="Laser power unsafe") -> ()  [unwired: 1 in, 1 out]
                }
              }
            }
          }
        }
      }
      event "Record Movie Button": Value Change {
        n210 = event-data() -> ()  [unwired: 1 in, 1 out]
        n211 = local read "Excitation"() -> (w345:T4)
        n212 = local read "Illumination:"() -> (w333:T2)
        n213 = local read "frame interval unit"() -> (w353:u32)
        n214 = local read "Acquisition Period"() -> (w352:dbl)
        n215 = for {
          tunnel: w345 -> [w359] mode=indexing
          tunnel: [w358] -> w344 mode=indexing
          n216 = Unbundle By Name(w359) -> ("Enable"=w358:bool)
        }
        n217 = local read "Illumination:"() -> (w340:T2)
        n218 = Equal?(x=w333, y=T2."Continuous") -> (x = y?=w332:bool)
        n219 = Equal?(x=w340, y=T2."Alternating") -> (x = y?=w338:bool)
        n220 = Boolean To (0,1)(Boolean=w344) -> (0, 1=w343:i16[])
        n221 = Multiply(x=w353, y=w352) -> (x*y=w351:dbl)
        n222 = Boolean To (0,1)(Boolean=w332) -> (0, 1=w331:i16)
        n223 = Add Array Elements(numeric array=w343) -> (sum=w342:i16)
        n224 = local write "Record Movie Button"(FALSE ("Record Movie Button")) -> ()
        n225 = Select(t=w342, s=w338, f=i16 1) -> (s? t:f=w337:i16)
        n226 = Build Path(base path="File Path:", name or relative path="File Name:") -> (appended path=w350:path)
        n227 = Multiply(x=w337, y="Frames:") -> (x*y=w335:dbl)
        n228 = Add(x=w335, y=w331) -> (x+y=w334:dbl)
        n229 = local read "current settings"() -> (w347:T1)
        n230 = Bundle By Name(cluster=w347, "fluidics trigger frame"="Trigger on frame number\n(set to zero to disable)", "Frames to Acquire"=w334, "Frames to Skip"=w331, "Exposure Time (ms)"=w351, "File Path"=w350) -> (w346:T1)
        n231 = local read "Active Cameras"() -> (w321:cluster{"Enable":bool, "Name":string}[])
        n232 = for {
          tunnel: w321 -> [w357] mode=indexing
          tunnel: [w356] -> w322 mode=indexing
          n233 = Unbundle By Name(w357) -> ("Enable"=w356:bool)
        }
        n234 = Bundle By Name(cluster=T17 {"Camera Settings"={"Exposure Time (ms)"=100.0, "Binning"=enum."2x2", "Scan Mode"=0, "Frames to Acquire"=1000.0, "Pixel Correction"=FALSE, "Frames to Skip"=0, "File Path"=path "", "Duty cycle"=0.0, "ALEX"=FALSE, "Shutter Enable"=[], "fluidics trigger frame"=0, "Bit Depth"=0, "Image Width (px)"=0, "Image Height (px)"=0, "Horizontal Offset (px)"=0, "Vertical Offset (px)"=0}, "Auto-Advance"=TRUE, "Auto Focus"=TRUE, "Injection Countdown"=TRUE, "Fields"=1, "Lanes"=1, "Acquisition type"=enum."Movie series"} ("Movie Series"), "Camera Settings"=w346, "Auto-Advance"="Auto-Advance", "Auto Focus"="Auto-Focus", "Injection Countdown"="Injection Countdown", "Fields"="Fields:", "Lanes"="Lanes:", "Acquisition type"="Acquisition type") -> (w324:T17)
        n235 = call "Send Set Enabled Cameras.vi"("Cameras Enabled"=w322, "Message Enqueuer"=w355) -> ("error out"=w319:errorcluster, "Message Enqueuer out"=w320:refnum<class "Message Enqueuer.lvclass">)  [unwired: 8 in]
        n236 = call "Send Start Recording.vi"("error in (no error)"=w319, "Movie Series"=w324, "Message Enqueuer"=w320) -> ()  [unwired: 7 in, 2 out]
      }
      event Value Change {
        n237 = event-data() -> ("NewVal"=w363:T3)  [unwired: 1 in, 5 out]
        n238 = Equal?(x=Movie_auto-numbering."Multi-lane series" ("y"), y=w363) -> (x = y?=w361:bool)
        n239 = Not Equal?(x=w363, y=Movie_auto-numbering."Single movie") -> (x != y?=w360:bool)
        n240 = property on="Lanes:" class="DigNum (strict)"("Visible"=w361) -> ()  [unwired: 2 in, 2 out]
        n241 = property on="Fields:" class="DigNum (strict)"("Visible"=w360) -> ()  [unwired: 2 in, 2 out]
        n242 = case shown="False" w361 {
          frame False {
            n243 = local write "Lanes:"(1 ("Fields:")) -> ()
          }
          frame True {
          }
        }
        n244 = local write "Auto-Advance"(w360) -> ()
        n245 = case shown="False" w360 {
          frame False {
            n246 = local write "Fields:"(1 ("Fields:")) -> ()
          }
          frame True {
          }
        }
      }
      event User Event {
        # "This event is triggered whenever the Application changes Mode,\nfor example when user clicks 'show live' or 'stream acquisition'.\nUse this to update the UI to reflect the current application state"
        n247 = event-data() -> ("Mode"=w367:T5)  [unwired: 1 in, 4 out]
        "Current Application Mode" <- w367
        n248 = case shown="\"Stream\"" w367 {
          frame "Idle", "Cancel" {
            w368 = T6."Enabled" ("Disabled")
            n249 = local write "Active Shutter Button"(FALSE ("Active Shutter Button")) -> ()
            n250 = property on="Live Viewer Start" class="Bool (strict)"("BoolText.Text"="Show Live" ("Boolean Text.Text")) -> ()  [unwired: 2 in, 2 out]
            n251 = property on="Record Movie Button" class="Bool (strict)"("DisabledEnum"=T6."Enabled" ("Disabled")) -> ()  [unwired: 2 in, 2 out]
            n252 = property on="Cancel Movie Button" class="Bool (strict)"("DisabledEnum"=T6."Disabled and Grayed Out" ("Disabled")) -> ()  [unwired: 2 in, 2 out]
            n253 = property on="Record Movie Button" class="Bool (strict)"("DisabledEnum"=w368) -> ()  [unwired: 2 in, 2 out]
            n254 = property on="Auto-focus" class="Bool"("DisabledEnum"=w368) -> ()  [unwired: 2 in, 2 out]
            n255 = property on="Camera Settings" class="TabCtl (strict)"("DisabledEnum"=w368) -> ()  [unwired: 2 in, 2 out]
            n256 = property on="Advanced Camera Settings" class="TabCtl (strict)"("DisabledEnum"=w368) -> ()  [unwired: 2 in, 2 out]
            n257 = property on="Stream Acquisition" class="TabCtl (strict)"("DisabledEnum"=w368) -> ()  [unwired: 2 in, 2 out]
            n258 = property on="Live Viewer Start" class="Bool (strict)"("DisabledEnum"=w368) -> ()  [unwired: 2 in, 2 out]
          }
          frame Default {
          }
          frame "Live" {
            w373 = T6."Disabled and Grayed Out" ("Disabled")
            n259 = property on="Live Viewer Start" class="Bool (strict)"("BoolText.Text"="Stop Live" ("Boolean Text.Text")) -> ()  [unwired: 2 in, 2 out]
            n260 = local write "Active Shutter Button"(TRUE ("Active Shutter Button")) -> ()
            n261 = property on="Record Movie Button" class="Bool (strict)"("DisabledEnum"=w373) -> ()  [unwired: 2 in, 2 out]
            n262 = property on="Camera Settings" class="TabCtl (strict)"("DisabledEnum"=w373) -> ()  [unwired: 2 in, 2 out]
            n263 = property on="Advanced Camera Settings" class="TabCtl (strict)"("DisabledEnum"=w373) -> ()  [unwired: 2 in, 2 out]
            n264 = property on="Auto-focus" class="Bool"("DisabledEnum"=w373) -> ()  [unwired: 2 in, 2 out]
          }
          frame "Stream" {
            w376 = T6."Disabled and Grayed Out" ("Disabled")
            n265 = local write "Active Shutter Button"(TRUE ("Active Shutter Button")) -> ()
            n266 = property on="Cancel Movie Button" class="Bool (strict)"("DisabledEnum"=T6."Enabled" ("Disabled")) -> ()  [unwired: 2 in, 2 out]
            n267 = property on="Auto-focus" class="Bool"("DisabledEnum"=w376) -> ()  [unwired: 2 in, 2 out]
            n268 = property on="Record Movie Button" class="Bool (strict)"("DisabledEnum"=w376) -> ()  [unwired: 2 in, 2 out]
            n269 = property on="Live Viewer Start" class="Bool (strict)"("DisabledEnum"=w376) -> ()  [unwired: 2 in, 2 out]
            n270 = property on="Camera Settings" class="TabCtl (strict)"("DisabledEnum"=w376) -> ()  [unwired: 2 in, 2 out]
            n271 = property on="Advanced Camera Settings" class="TabCtl (strict)"("DisabledEnum"=w376) -> ()  [unwired: 2 in, 2 out]
            n272 = property on="Stream Acquisition" class="TabCtl (strict)"("DisabledEnum"=w376) -> ()  [unwired: 2 in, 2 out]
          }
          frame "Autofocus" {
            w379 = T6."Disabled and Grayed Out" ("Disabled")
            n273 = property on="Record Movie Button" class="Bool (strict)"("DisabledEnum"=w379) -> ()  [unwired: 2 in, 2 out]
            n274 = property on="Live Viewer Start" class="Bool (strict)"("DisabledEnum"=w379) -> ()  [unwired: 2 in, 2 out]
            n275 = property on="Advanced Camera Settings" class="TabCtl (strict)"("DisabledEnum"=w379) -> ()  [unwired: 2 in, 2 out]
            n276 = property on="Camera Settings" class="TabCtl (strict)"("DisabledEnum"=w379) -> ()  [unwired: 2 in, 2 out]
            n277 = property on="Auto-focus" class="Bool"("DisabledEnum"=w379) -> ()  [unwired: 2 in, 2 out]
            n278 = property on="Cancel Movie Button" class="Bool (strict)"("DisabledEnum"=T6."Enabled" ("Disabled")) -> ()  [unwired: 2 in, 2 out]
          }
        }
      }
      event "Cancel Movie Button": Value Change {
        n279 = event-data() -> ()  [unwired: 1 in, 6 out]
        n280 = Two Button Dialog(message="Cancel acquisition?", 1:"No, continue acquisition" ("F button name (\"Cancel\")"), 2:"Yes, cancel" ("T button name (\"OK\")")) -> (T button?=w385:bool)
        n281 = case shown="True" w385 {
          tunnel: w381 -> [_ w386]
          frame False {
          }
          frame True {
            n282 = call "Send Cancel Operation.vi"("Message Enqueuer"=w386) -> ()  [unwired: 9 in, 2 out]
          }
        }
      }
      event "Illumination:": Value Change {
        # "This will trigger the event case\nto update number of lines etc."
        n283 = event-data() -> ()  [unwired: 1 in, 4 out]
        n284 = local read "Exposure (ms)"() -> (w390:dbl)
        n285 = local read "Duty Cycle:"() -> (w389:dbl)
        n286 = Greater Than 0?(x="Illumination:") -> (x > 0?=w387:bool)
        n287 = case shown="True" w387 {
          tunnel: w390 -> [w395 w399]
          tunnel: [w393 w398] -> w392
          tunnel: w389 -> [_ w397]
          frame False {
            w394 = T6."Disabled and Grayed Out" ("Disabled")
            w396 = u16 1 items=["ms"=1, "s"=1000, "min"=60000] ("frame interval unit")
            # "Strobe  -> standard mode"
            n288 = property on="Acquisition Period" class="DigNum (strict)"("DisabledEnum"=w394, "Value"=w395) -> (error out=w393:errorcluster)  [unwired: 2 in, 1 out]
            n289 = property on="frame interval unit" class="Ring (strict)"("DisabledEnum"=w394, "Value"=w396) -> ()  [unwired: 2 in, 2 out]
          }
          frame True {
            w403 = T6."Enabled" ("Disabled")
            # "Standard -> strobe mode"
            n290 = Divide(x=w399, y=w397) -> (x/y=w400:dbl)
            n291 = formula code="units=1;\nif (exposure>=1000) {\n    units=1000;\n}\nif (exposure>=60000) {\n    units=60000;\n}\ninterval = exposure/units;"("exposure"=w400) -> ("interval"=w401:dbl, "units"=w402:dbl)
            n292 = property on="Acquisition Period" class="DigNum (strict)"("DisabledEnum"=w403, "Value"=w401) -> (error out=w398:errorcluster)  [unwired: 2 in, 1 out]
            n293 = property on="frame interval unit" class="Ring (strict)"("DisabledEnum"=w403, "Value"=w402) -> ()  [unwired: 2 in, 2 out]
          }
        }
        n294 = local read "Pixel Correction"() -> (w391:enum16{"Live Only", "On", "Off"})
        n295 = property on="Pixel Correction" class="Enum (strict)"(error in=w392, "Val(Sgnl)"=w391) -> ()  [unwired: 1 in, 2 out]
      }
      event "Exposure (ms)": Value Change {
        # "trigger event case to update other controls"
        n296 = event-data() -> ("NewVal"=w405:dbl, "CtlRef"=w409:refnum<vi>)  [unwired: 1 in]
        n297 = local read "Illumination:"() -> (w404:T2)
        n298 = case shown="\"Stroboscopic\", \"Alternating\"" w404 {
          tunnel: w405 -> [w411 w420]
          tunnel: [w410 w416] -> w408
          frame "Continuous", Default {
            n299 = In Range and Coerce(upper limit=10000.0, x=w411, lower limit=0.1) -> (coerced(x)=w410:dbl)  [unwired: 1 out]
            n300 = local write "Acquisition Period"(w410) -> ()
          }
          frame "Stroboscopic", "Alternating" {
            w419 = 2.0  # shutter min exposure (ms)
            n301 = local read "Acquisition Period"() -> (w414:dbl)
            n302 = local read "frame interval unit"() -> (w418:u32)
            n303 = Multiply(x=w414, y=w418) -> (x*y=w415:dbl)
            n304 = In Range and Coerce(upper limit=w415, x=w420, lower limit=w419) -> (coerced(x)=w416:dbl)  [unwired: 1 out]
            n305 = Divide(x=w416, y=w415) -> (x/y=→"Duty Cycle:":dbl)
          }
        }
        n306 = property class="DigNum (strict)"(reference=w409, "Value"=w408) -> (error out=w406:errorcluster)  [unwired: 1 in, 1 out]
        n307 = local read "Pixel Correction"() -> (w407:enum16{"Live Only", "On", "Off"})
        n308 = property on="Pixel Correction" class="Enum (strict)"(error in=w406, "Val(Sgnl)"=w407) -> ()  [unwired: 1 in, 2 out]
      }
      event "Acquisition Period": Value Change {
        # "trigger event case to update other controls"
        n309 = event-data() -> ("CtlRef"=w429:refnum<vi>, "NewVal"=w426:dbl)  [unwired: 1 in, 4 out]
        n310 = local read "frame interval unit"() -> (w424:u32)
        n311 = local read "Exposure (ms)"() -> (w423:dbl)
        n312 = Multiply(x=w426, y=w424) -> (x*y=w421:dbl)
        n313 = Divide(x=w421, y=w424) -> (x/y=w425:dbl)
        n314 = Divide(x=w423, y=w421) -> (x/y=w422:dbl)
        n315 = property class="DigNum (strict)"(reference=w429, "Value"=w425) -> (error out=w428:errorcluster)  [unwired: 1 in, 1 out]
        n316 = local write "Duty Cycle:"(w422) -> ()
        n317 = local read "Pixel Correction"() -> (w427:enum16{"Live Only", "On", "Off"})
        n318 = property on="Pixel Correction" class="Enum (strict)"(error in=w428, "Val(Sgnl)"=w427) -> ()  [unwired: 1 in, 2 out]
      }
      event "Auto-focus": Value Change {
        n319 = event-data() -> ()  [unwired: 1 in, 1 out]
        n320 = for {
          tunnel: "Active Cameras" -> [w437] mode=indexing
          tunnel: [w436] -> w434 mode=indexing
          n321 = Unbundle By Name(w437) -> ("Enable"=w436:bool)
        }
        n322 = call "Send Set Enabled Cameras.vi"("Cameras Enabled"=w434, "Message Enqueuer"=w433) -> ("error out"=w431:errorcluster, "Message Enqueuer out"=w432:refnum<class "Message Enqueuer.lvclass">)  [unwired: 8 in]
        n323 = local read "current settings"() -> (w435:T1)
        n324 = call "Send Start Autofocus.vi"("error in (no error)"=w431, "Camera Settings"=w435, "Message Enqueuer"=w432) -> ()  [unwired: 7 in, 2 out]
      }
      event "Enforce software stage limits", "Forward step (mm)", "Lane separation (mm)": Value Change {
        n325 = event-data() -> ()  [unwired: 1 in, 1 out]
        n326 = call "Send Stage Enforce Limits.vi"("Lane separation (mm)"="Lane separation (mm)", "Forward step (mm)"="Forward step (mm)", "Enforce software stage limits"="Enforce software stage limits", "Message Enqueuer"=w441) -> ()  [unwired: 6 in, 2 out]
      }
      event "Calibrate Polarizer": Value Change {
        n327 = event-data() -> ()  [unwired: 1 in, 1 out]
        n328 = call "Send Calibrate Polarizer.vi"("Message Enqueuer"=w442) -> ()  [unwired: 9 in, 2 out]
      }
    }
  }
  n329 = call-parent "Actor Core.vi"("error in"=w8, "Actor in"=w7) -> ("error out"=w1:errorcluster, "Actor out"=w3:refnum<class "Actor.lvclass">)  [unwired: 8 in]
  n330 = flat-sequence {
    tunnel: [w445] -> w4
    tunnel: w3 -> [w445]
    tunnel: [w444] -> w2
    tunnel: w1 -> [w444]
    frame #0 {
      n331 = local write "Stop Button"(TRUE ("Stop Button")) -> ()
    }
  }
  n332 = Unregister For Events(event registration refnum=w9) -> ()  [unwired: 1 in, 1 out]
  "error out" <- w2
  "Actor out" <- w4
